vi "Logger_JSON.vi"(8 "error in":errorcluster, 10 "General_Info":T1, 11 "appended array":string[](array[string])) -> (0 "error out":errorcluster)   [LabVIEW 2023]
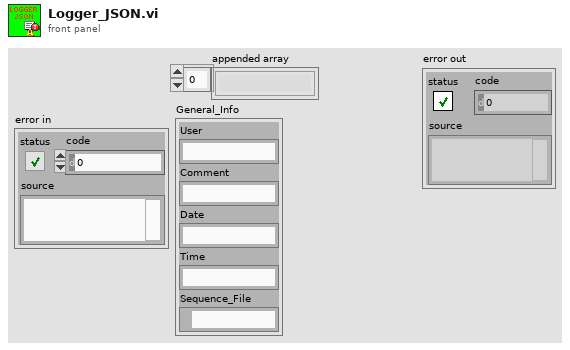
[diagram p1: front panel]
types:
  T1 = cluster{"User":string, "Comment":string, "Date":string, "Time":string, "Sequence_File":path}
  T2 = enum16{"open", "replace", "create", "open or create", "replace or create", "replace or create with confirmation"}
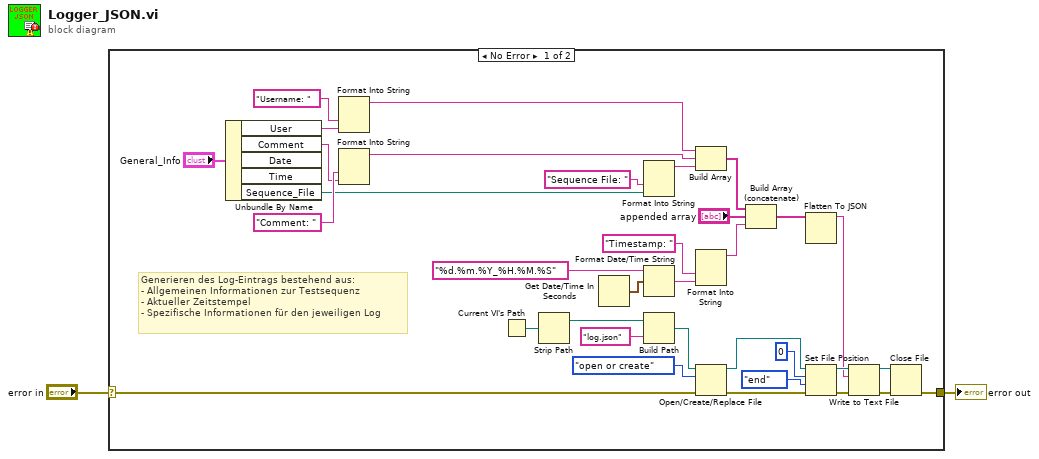
[diagram p0: block diagram]
diagram:
  n1 = case shown="No Error" "error in" {
    selector: "error in" -> [w3 w37]
    tunnel: [w22 w37] -> w2
    frame No Error {
      # "Generieren des Log-Eintrags bestehend aus:\n- Allgemeinen Informationen zur Testsequenz\n- Aktueller Zeitstempel\n- Spezifische Informationen für den jeweiligen Log"
      n2 = Unbundle By Name("General_Info") -> ("User"=w12:string, "Comment"=w10:string, "Sequence_File"=w8:path)  [unwired: 2 out]
      n3 = Format Into String("Username: ", w12) -> (resulting string=w7:string)  [unwired: 3 in, 1 out]
      n4 = Format Into String("Comment: ", w10) -> (resulting string=w6:string)  [unwired: 3 in, 1 out]
      n5 = Current VI's Path() -> (path=w35:path)
      n6 = Strip Path(path=w35) -> (stripped path=w34:path)  [unwired: 1 out]
      n7 = Get Date/Time In Seconds() -> (seconds since 1Jan1904=w21:timestamp)
      n8 = Format Into String("Sequence File: ", w8) -> (resulting string=w5:string)  [unwired: 3 in, 1 out]
      n9 = Format Date/Time String(time format string (%c)="%d.%m.%Y_%H.%M.%S", seconds (now)=w21) -> (date/time string=w19:string)  [unwired: 1 in]
      n10 = Build Path(base path=w34, name or relative path="log.json") -> (appended path=w33:path)
      n11 = Build Array(w7, w6, w5) -> (w4:string[])
      n12 = Format Into String("Timestamp: ", w19) -> (resulting string=w17:string)  [unwired: 3 in, 1 out]
      n13 = Open/Create/Replace File(file path (use dialog)=w33, error in=w3, operation (0:open)=T2."open or create") -> (refnum out=w31:refnum<file>, error out=w30:errorcluster)  [unwired: 3 in, 1 out]
      n14 = Build Array (concatenate)(w4, "appended array", w17) -> (w16:string[])
      n15 = Flatten To JSON(anything=w16) -> (JSON string=w24:string)  [unwired: 2 in, 1 out]
      n16 = Set File Position(offset (in bytes) (0)=i64 0, refnum=w31, from (0:start)=enum16{"start", "end", "current"}."end", error in=w30) -> (refnum out=w26:refnum<file>, error out=w29:errorcluster)
      n17 = Write to Text File(file (use dialog)=w26, text=w24, error in=w29) -> (refnum out=w27:refnum<file>, error out=w28:errorcluster)  [unwired: 1 in, 1 out]
      n18 = Close File(refnum=w27, error in=w28) -> (error out=w22:errorcluster)  [unwired: 1 out]
    }
    frame Error {
    }
  }
  "error out" <- w2
